vi "10.1.vi"() -> ()   [LabVIEW 2017]
panel:
  out "4":bool
  out "3":bool
  out "2":bool
  out "1":bool
  out "0":bool
  in  "stop":bool
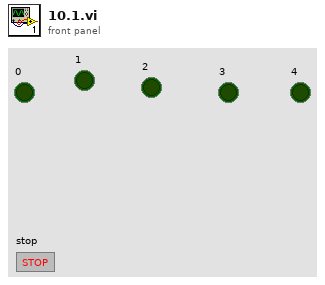
[diagram p1: front panel]
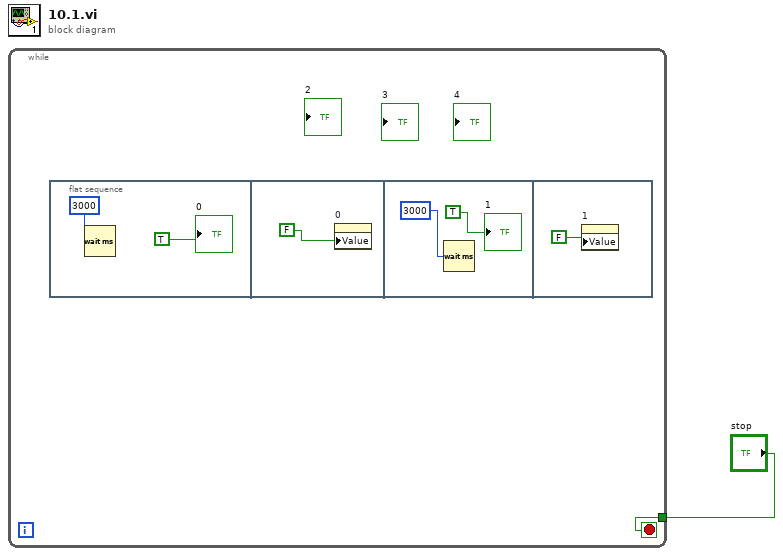
[diagram p0: block diagram]
diagram:
  n1 = while {
    tunnel: "stop" -> [w2]
    stop <- w2 stop-if-true
    n2 = flat-sequence {
      frame #0 {
        n3 = Wait (ms)(milliseconds to wait=3000) -> ()  [unwired: 1 out]
        "0" <- TRUE
      }
      frame #1 {
        n4 = property on="0" class="Bool (strict)"("Value"=FALSE) -> ()  [unwired: 2 in, 2 out]
      }
      frame #2 {
        n5 = Wait (ms)(milliseconds to wait=3000) -> ()  [unwired: 1 out]
        "1" <- TRUE
      }
      frame #3 {
        n6 = property on="1" class="Bool (strict)"("Value"=FALSE) -> ()  [unwired: 2 in, 2 out]
      }
    }
  }
